vi "LVClass_CorrectionDataManager CheckRelativePositionsSaturation.vi"(0 "CorrectionDataManager in":refnum<class "CorrectionDataManager.lvclass">, 5 "Deltaposition":sgl[](array[numeric]), 7 "position":sgl[](array[numeric]), 11 "error in (no error)":errorcluster) -> (4 "CorrectionDataManager out":refnum<class "CorrectionDataManager.lvclass">, 10 "saturated_act_count":i32, 15 "error out":errorcluster)   [LabVIEW 2020, in "CorrectionDataManager.lvclass"]
doc: "Simulation of the expected slopes given the Wavefront corrector preferences\nand an array of positions.\n\n--------------------------------------------------------------------------------\n\n<B>corrdata_managerIn </B> : CorrDataManager object.\n<B>corrdata_managerOut </B> : CorrDataManager object.\n<B>min </B> : WavefrontCorrector preferences : lowest command value.\n<B>max </B> : WavefrontCorrector preferences : highest command value.\n<B>validity </B> : WavefrontCorrector preferences : status.\n<B>fixed_values </B> : WavefrontCorrector preferences : fixed positions.\n<B>positions </B> : Array of size actuators count, containing for each actuator its current\n position.\n<B>HasoSlopes </B> : HasoSlopes object, where the simulated slopes are stored.\n<B>ErrorIn </B> : Error\n<B>ErrorOut </B> : Error\n\n--------------------------------------------------------------------------------"
uses:
  CorrectionDataManager.lvclass
  CorrectionDataManager.lvclass/CorrectionDataManager.ctl
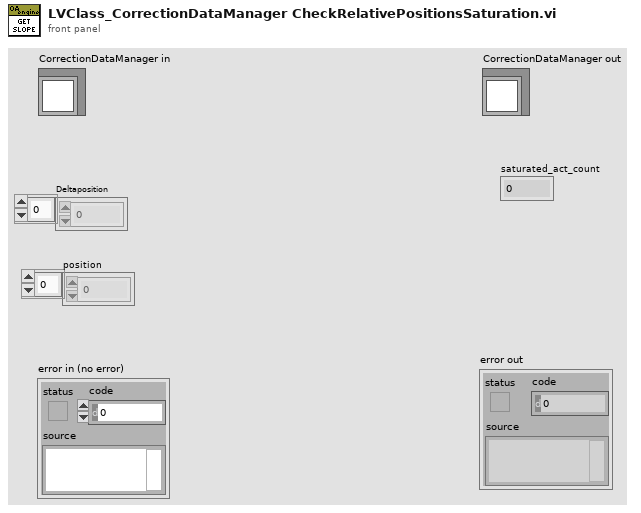
[diagram p1: front panel]
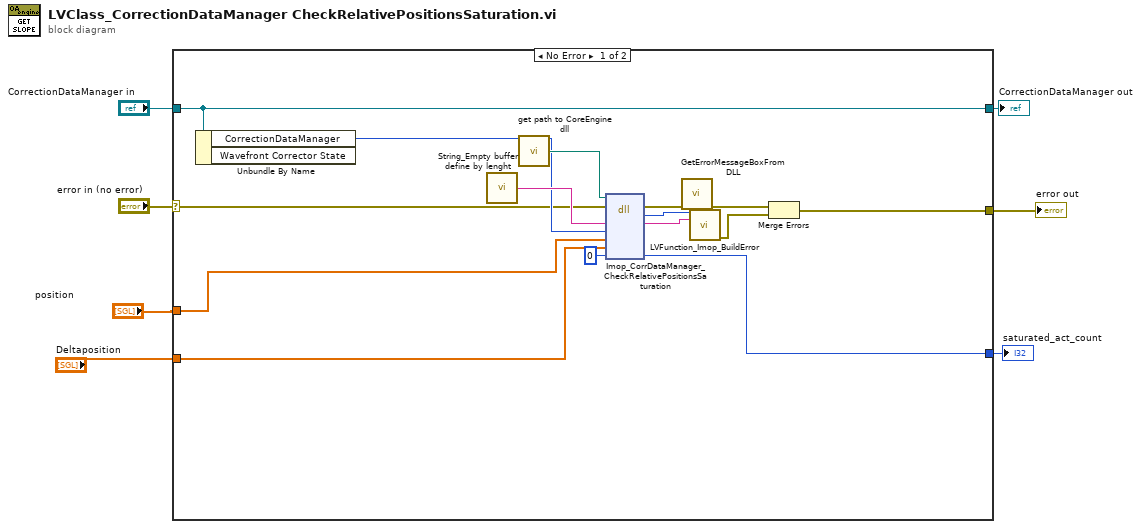
[diagram p0: block diagram]
diagram:
  n1 = case shown="No Error" "error in (no error)" {
    selector: "error in (no error)" -> [w12 w24]
    tunnel: [w20 w24] -> w5
    tunnel: [w19 w23] -> w4
    tunnel: "CorrectionDataManager in" -> [w19 w23]
    tunnel: "position" -> [w11 _]
    tunnel: [w8 _] -> w1
    tunnel: "Deltaposition" -> [w10 _]
    frame No Error {
      n2 = Unbundle By Name(w19) -> ("CorrectionDataManager"=w13:i32)  [unwired: 1 out]
      n3 = call "String_Empty buffer define by lenght.vi"() -> ("Empty buffer"=w17:string)  [unwired: 1 in]
      n4 = call "get path to CoreEngine dll.vi"() -> ("path to c_interface_vc100.dll"=w18:path)  [unwired: 12 in, 3 out]
      n5 = dll-call lib="D:/soft/HASO_v3/SVN_trunk/ImOpCoreEngine4_LV2011/DLLs/c_interface_vc100.dll" fn="Imop_CorrDataManager_CheckRelativePositionsSaturation"(path in=w18, error in=w12, "message"=w17, "WavefrontCorrection"=w13, "current position"=w11, "delta position"=w10, "saturated_act_count"=0) -> (error out=w16:errorcluster, "return type"=w15:i32, "message"=w14:string, "saturated_act_count"=w8:i32)  [unwired: 4 in, 1 out]
      n6 = call "GetErrorMessageBoxFromDLL.vi"("error IN"=w16) -> ("error OUT"=w22:errorcluster)  [unwired: 10 in]
      n7 = call "LVFunction_Imop_BuildError.vi"("code"=w15, "String to Prepend to source (\"\")"=w14) -> ("error out"=w21:errorcluster)  [unwired: 13 in]
      n8 = Merge Errors(w22, w21) -> (w20:errorcluster)
    }
    frame Error {
    }
  }
  "error out" <- w5
  "CorrectionDataManager out" <- w4
  "saturated_act_count" <- w1
